vi "test_poliline.vi"() -> ()   [LabVIEW 2020]
panel:
  out "Image 2":T1(plugin-control)
  out "ROI":T2
  in  "stop":bool
  out "Image":T1(plugin-control)
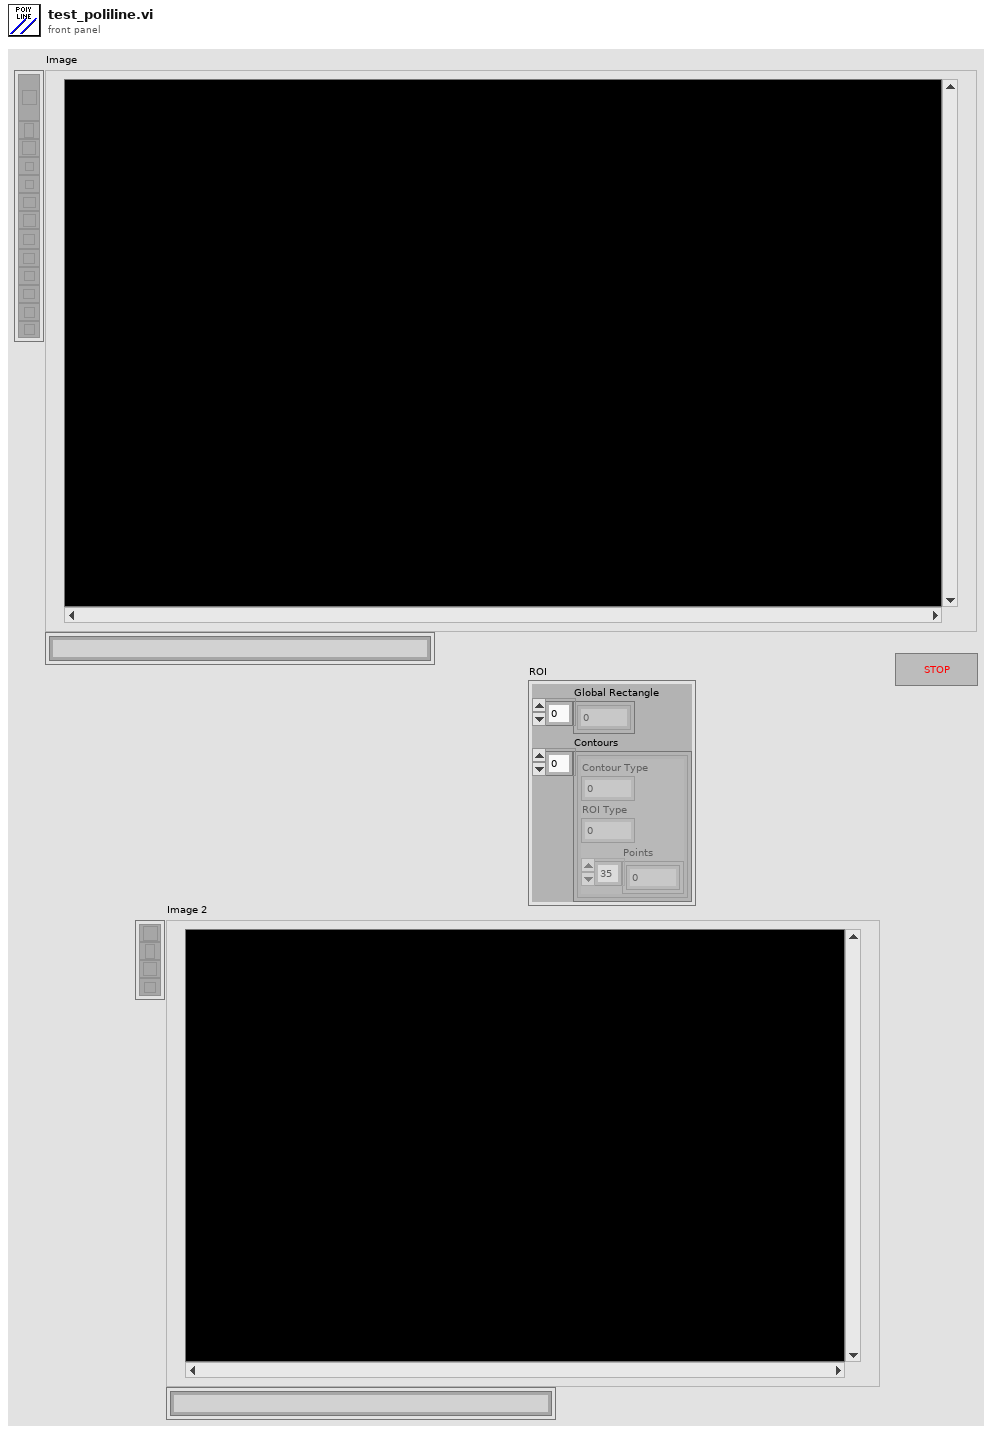
[diagram p1: front panel]
types:
  T1 = typedef "IMAQ Image.ctl" = refnum<image>
  T2 = cluster{"Global Rectangle":i32[], "Contours":cluster{"Contour Type":u32, "ROI Type":u32, "Points":i32[]}[]}
  T3 = typedef "Image Type" = u32
  T4 = cluster{"Zoom Tool":bool, "Selection Tool":bool, "Pan Tool":bool, "Point Tool":bool, "Line Tool":bool, "Rectangle Tool":bool, "Rotated Rectangle Tool":bool, "Polyline Tool":bool, "Polygon Tool":bool, "Freehand Tool":bool, "Closed Freehand Tool":bool, "Ellipse Tool":bool, "Annulus Tool":bool}
  T5 = cluster{"Contour Type":u32, "ROI Type":u32, "Points":i32[]}[]
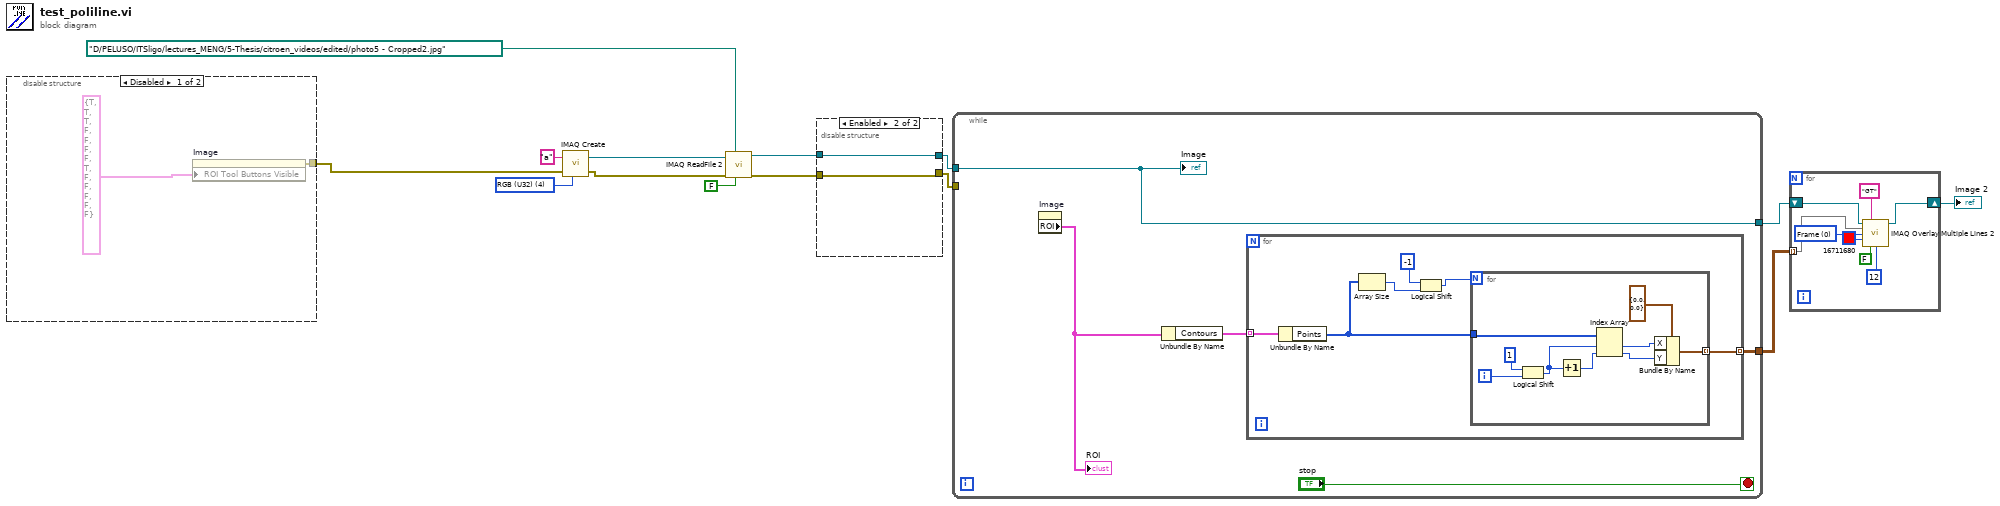
[diagram p0: block diagram]
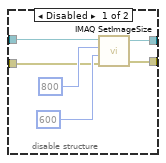
[diagram p3: hidden frame]
diagram:
  w13 = T3 4 items=["Grayscale (U8)", "Grayscale (I16)", "Grayscale (SGL)", "Complex (CSG)", "RGB (U32)", "HSL (U32)", "RGB (U64)", "Grayscale (U16)"] ("Image Type")
  n1 = disable-structure shown="Disabled" {
    disable-tunnel: [w16 _] -> w5
    frame Disabled {
      n2 = property on="Image" class="ImageControl"("ROI Tool Buttons Visible"=T4 {"Zoom Tool"=TRUE, "Selection Tool"=TRUE, "Pan Tool"=TRUE, "Point Tool"=FALSE, "Line Tool"=FALSE, "Rectangle Tool"=FALSE, "Rotated Rectangle Tool"=FALSE, "Polyline Tool"=TRUE, "Polygon Tool"=FALSE, "Freehand Tool"=FALSE, "Closed Freehand Tool"=FALSE, "Ellipse Tool"=FALSE, "Annulus Tool"=FALSE} ("ROI Tool Buttons Visible:All Elements")) -> (error out=w16:errorcluster)  [unwired: 2 in, 1 out]
    }
    frame Enabled {
    }
  }
  n3 = call "IMAQ Create"("Image Name"="a", "Image Type"=w13, "error in (no error)"=w5) -> ("New Image"=w8:T1, "error out"=w12:errorcluster)  [unwired: 2 in]
  n4 = call "IMAQ ReadFile 2"("Use File Path Image Type"=FALSE, "File Path"=path "D:/PELUSO/ITSligo/lectures_MENG/5-Thesis/citroen_videos/edited/photo5 - Cropped2.jpg" ("name or relative path"), "error in (no error)"=w12, "Image"=w8) -> ("error out"=w9:errorcluster, "Image Out"=w7:T1)  [unwired: 3 in, 3 out]
  n5 = disable-structure shown="Enabled" {
    disable-tunnel: [w22 w24] -> w11
    disable-tunnel: [w21 w23] -> w10
    disable-tunnel: w9 -> [w18 w24]
    disable-tunnel: w7 -> [w17 w23]
    frame Disabled {
      n6 = call "IMAQ SetImageSize"("error in (no error)"=w18, "Y Resolution"=600 ("X Resolution"), "X Resolution"=800, "Image"=w17) -> ("error out"=w22:errorcluster, "Image Out"=w21:T1)  [unwired: 1 in]
    }
    frame Enabled {
    }
  }
  n7 = while {
    tunnel: w11 -> [_]
    tunnel: w10 -> [w28]
    tunnel: [w28] -> w4
    tunnel: [w25] -> w2
    stop <- "stop" stop-if-true
    n8 = property on="Image" class="ImageControl"() -> ("ROI"=w27:T2)  [unwired: 2 in, 2 out]
    "ROI" <- w27
    n9 = Unbundle By Name(w27) -> ("Contours"=w26:T5)
    n10 = for {
      tunnel: w26 -> [w35] mode=indexing
      tunnel: [w30] -> w25 mode=indexing
      n11 = Unbundle By Name(w35) -> ("Points"=w34:i32[])
      n12 = Array Size(array=w34) -> (size(s)=w33:i32)
      n13 = Logical Shift(y=-1 ("x"), x=w33) -> (x << y=w32:i32)
      n14 = for {
        N: w32 -> [_]
        tunnel: w34 -> [w44]
        tunnel: [w36] -> w30 mode=indexing
        i -> [w41]
        n15 = Logical Shift(y=1 ("x"), x=w41) -> (x << y=w40:i32)
        n16 = Increment(x=w40) -> (x+1=w43:i32)
        n17 = Index Array(array=w44, index #1=w40, index #2=w43) -> (element #1=w38:i32, element #2=w37:i32)
        n18 = Bundle By Name(cluster=cluster{"X":dbl, "Y":dbl} {"X"=0.0, "Y"=0.0} ("Point Coordinates"), "X"=w38, "Y"=w37) -> (w36:cluster{"X":dbl, "Y":dbl})
      }
    }
    "Image" <- w28
  }
  n19 = for {
    shift-right: [w51] -> w3
    shift-left: w4 -> [w52]
    tunnel: w2 -> [w46] mode=indexing
    w50 = u32 0 items=["Frame", "Fill"] ("Drawing Mode (Frame)")
    n20 = call "IMAQ Overlay Multiple Lines 2"("Image"=w52, "Group"="GT", "Line End Points"=w46, "Drawing Mode (Frame)"=w50, "Color"=u32 16711680, "Maintain Width?"=FALSE, "Width"=u32 12) -> ("Image Out"=w51:T1)  [unwired: 7 in, 1 out]
  }
  "Image 2" <- w3
